vi "Untitled 4.vi"   [LabVIEW 2017]
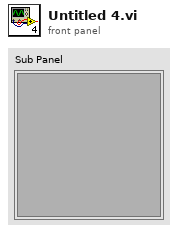
[diagram p1: front panel]
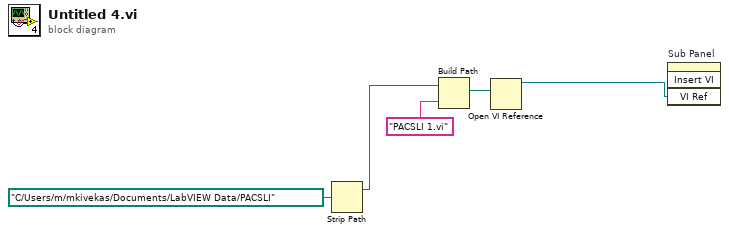
[diagram p0: block diagram]
diagram:
  n1 = Strip Path(path=path "C:/Users/m/mkivekas/Documents/LabVIEW Data/PACSLI") -> (stripped path=w3:path)  [unwired: 1 out]
  n2 = Build Path(base path=w3, name or relative path="PACSLI 1.vi") -> (appended path=w5:path)
  n3 = Open VI Reference(vi path=w5) -> (vi reference=w2:refnum<vi>)  [unwired: 5 in, 1 out]
  n4 = invoke on="Sub Panel" class="SubPnl" method="Insert VI"("VI Ref"=w2) -> ()  [unwired: 3 in, 4 out]
